vi "Digital_IO_Bit_Toggle.vi"(11 "lines":tag) -> (3 "Boolean":bool)   [LabVIEW 2017]
uses:
  <vilib>/DAQmx/read.llb/DAQmx Read (Digital Bool 1Line 1Point).vi
  <vilib>/DAQmx/write.llb/DAQmx Write (Digital Bool 1Line 1Point).vi
  <vilib>/DAQmx/create/channels.llb/DAQmx Create Channel (DO-Digital Output).vi
  <vilib>/DAQmx/miscellaneous.llb/DAQmx Fill In Error Info.vi
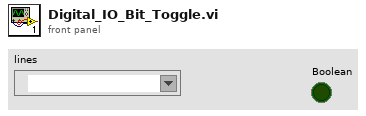
[diagram p1: front panel]
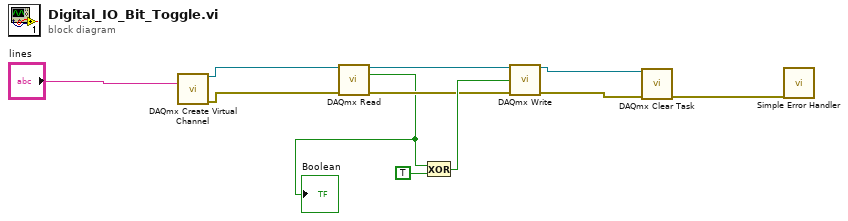
[diagram p0: block diagram]
diagram:
  n1 = call-poly <vilib>:"DAQmx Create Virtual Channel.vi"("lines"="lines") -> ("task out"=w9:refnum<k21>, "error out"=w6:errorcluster)  [unwired: 13 in]
  n2 = call-poly <vilib>:"DAQmx Read.vi"("task/channels in"=w9, "error in"=w6) -> ("task out"=w8:refnum<k21>, "data"=w1:bool, "error out"=w5:errorcluster)  [unwired: 11 in]
  "Boolean" <- w1
  n3 = Exclusive Or(1:TRUE ("y"), 2:w1) -> (0:w10:bool)
  n4 = call-poly <vilib>:"DAQmx Write.vi"("task/channels in"=w8, "data"=w10, "error in"=w5) -> ("task out"=w7:refnum<k21>, "error out"=w4:errorcluster)  [unwired: 10 in, 1 out]
  n5 = call <vilib>:"DAQmx Clear Task.vi"("task in"=w7, "error in"=w4) -> ("error out"=w3:errorcluster)  [unwired: 13 in]
  n6 = call <vilib>:"Simple Error Handler.vi"("error in (no error)"=w3) -> ()  [unwired: 4 in, 5 out]
